vi "BWC_MakeMasks.vi"() -> ()   [LabVIEW 2017]
uses:
  <vilib>/Utility/miscctls.llb/LVPoint32TypeDef.ctl
  <vilib>/Utility/miscctls.llb/LVPositionTypeDef.ctl
panel:
  in  "stop":bool
  in  "fill?(F)":bool
  in  "radius 2":i16
  out "Mouseclick Coords":T1
  out "Box Coords":T2
  out "Clicked Coords":T1
  out "new picture":picture
  in  "Path":path
  # "NOTE, must be a 24 bit color image to load properly at the moment."
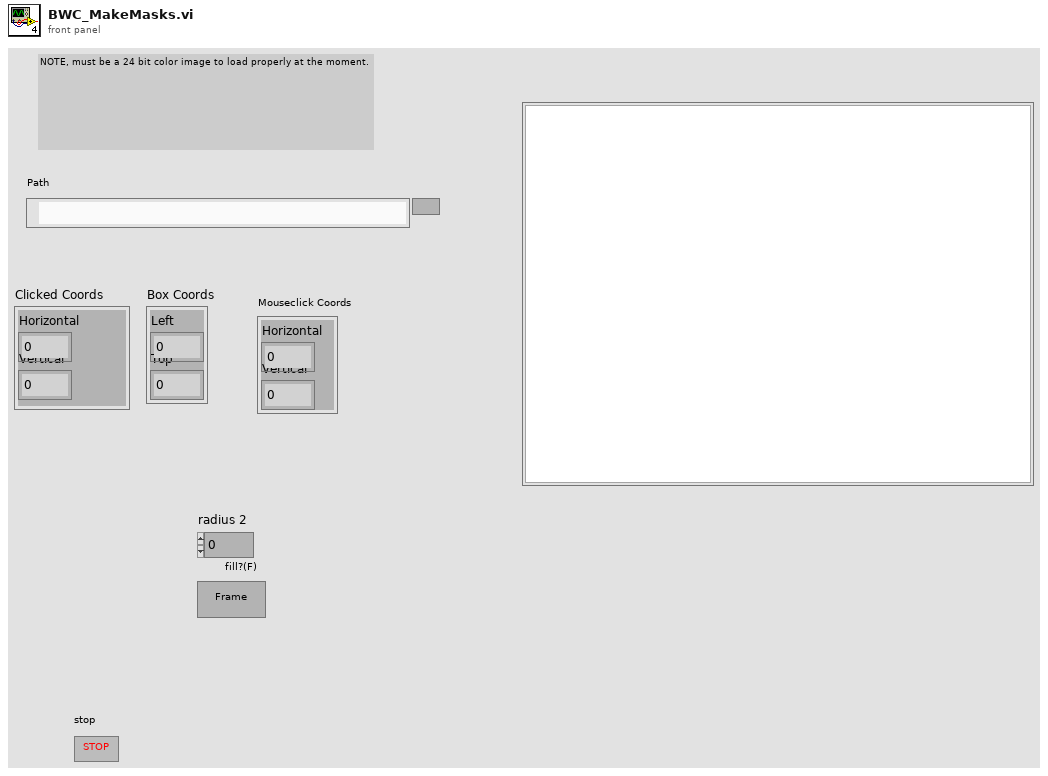
[diagram p1: front panel]
types:
  T1 = typedef "LVPoint32TypeDef.ctl" = cluster{"Horizontal":i32, "Vertical":i32}
  T2 = typedef "LVPositionTypeDef.ctl" = cluster{"Left":i32, "Top":i32}
  T3 = typedef "imagedata.ctl" = cluster{"image type":i32, "image depth":i32, "image":u8[], "mask":u8[], "colors":u32[], "Rectangle":cluster{"left":i16, "top":i16, "right":i16, "bottom":i16}}
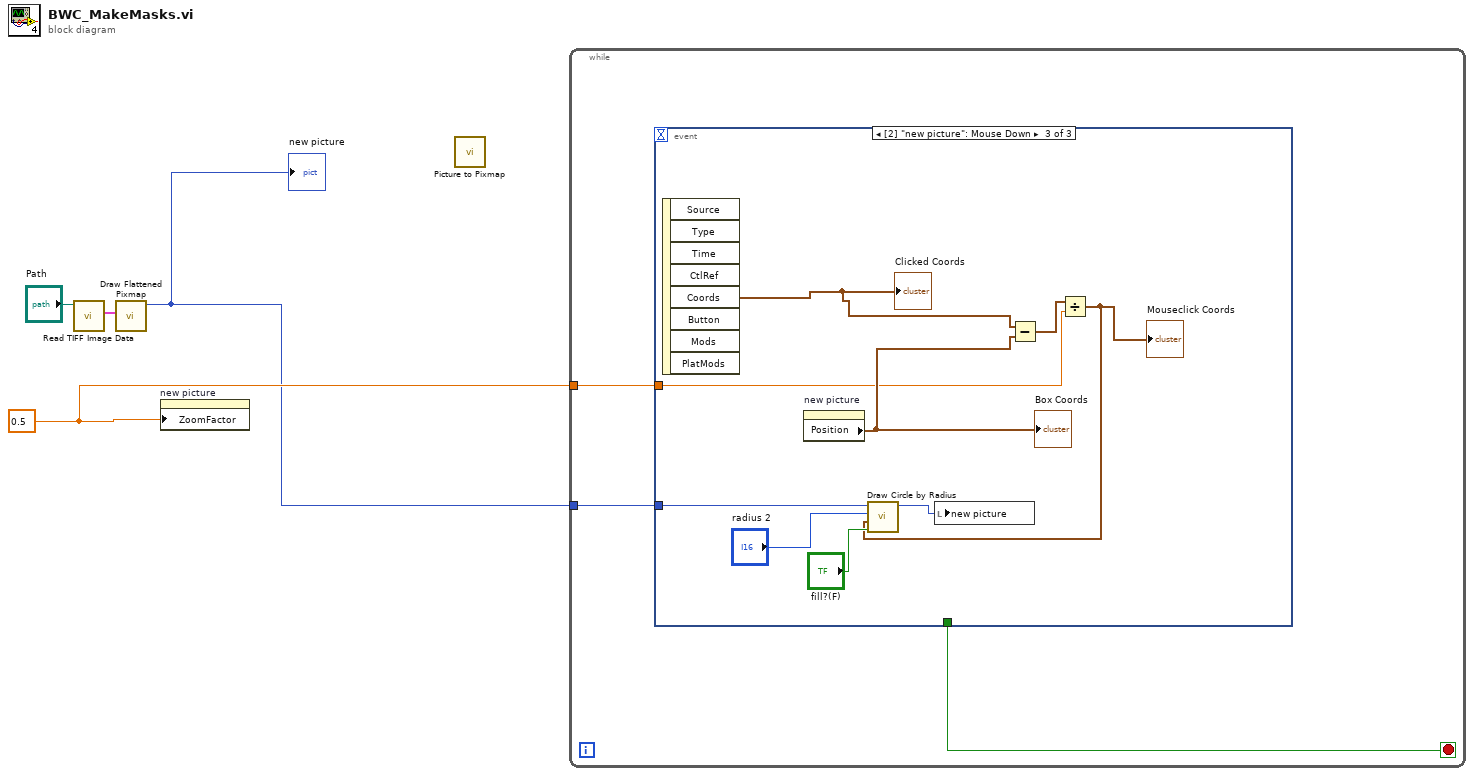
[diagram p0: block diagram]
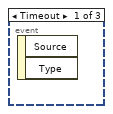
[diagram p2: hidden frame]
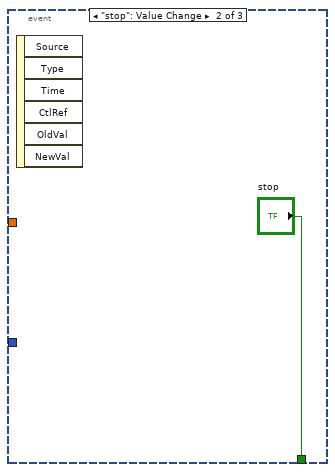
[diagram p3: hidden frame]
diagram:
  w2 = sgl 0.5 ("Zoom Factor")
  n1 = call "Read TIFF Image Data.vi"("path to TIFF file"="Path") -> ("image data"=w3:T3)  [unwired: 6 in, 2 out]
  n2 = call <vilib>:"Draw Flattened Pixmap.vi"("image data"=w3) -> ("new picture"=w1:picture)  [unwired: 8 in]
  "new picture" <- w1
  n3 = property on="new picture" class="Pict"("ZoomFactor"=w2) -> ()  [unwired: 2 in, 2 out]
  n4 = call <vilib>:"Picture to Pixmap.vi"() -> ()  [unwired: 10 in, 2 out]
  n5 = while {
    tunnel: w2 -> [w7]
    tunnel: w1 -> [w6]
    stop <- w5 stop-if-true
    n6 = event shown="[2] \"new picture\": Mouse Down" {
      selector: _ -> [_ _ _]
      dyn-events: _ -> [_ _ _]
      timeout: _ -> [_ _ _]
      tunnel: w7 -> [_ _ w15]
      tunnel: w6 -> [_ _ w14]
      tunnel: [_ "stop" _] -> w5
      event Timeout {
        n7 = event-data() -> ()  [unwired: 1 in, 2 out]
      }
      event "stop": Value Change {
        n8 = event-data() -> ()  [unwired: 1 in, 6 out]
      }
      event "new picture": Mouse Down {
        n9 = event-data() -> ("Coords"=w17:T1)  [unwired: 1 in, 7 out]
        "Clicked Coords" <- w17
        n10 = property on="new picture" class="Pict"() -> ("Position"=w16:T2)  [unwired: 2 in, 2 out]
        "Box Coords" <- w16
        n11 = Subtract(x=w17, y=w16) -> (x-y=w12:T1)
        n12 = Divide(x=w12, y=w15) -> (x/y=w9:cluster{"Horizontal":sgl, "Vertical":sgl})
        "Mouseclick Coords" <- w9
        n13 = call <vilib>:"Draw Circle by Radius.vi"("fill?(F)"="fill?(F)", "pixel center"=w9, "radius"="radius 2", "picture"=w14) -> ("new picture"=w10:picture)  [unwired: 7 in]
        n14 = local write "new picture"(w10) -> ()
      }
    }
  }
